vi "Create from Agent.vi"(8 "Error In":errorcluster, 11 "Agent In":refnum<class "Agent.lvclass">) -> (0 "Error Out":errorcluster, 2 "Identity":refnum<class "Agent Identity.lvclass">, 3 "Agent Out":refnum<class "Agent.lvclass">)   [LabVIEW 2018, in "Toolkit.lvlib" / "Agent Identity.lvclass"]
uses:
  Agent Identity.lvclass
  Agent/Agent.lvclass
  Agent/Agent.lvclass/Agent.ctl
  Session/Session.lvclass/Session.ctl
  SSH/SSH.lvclass
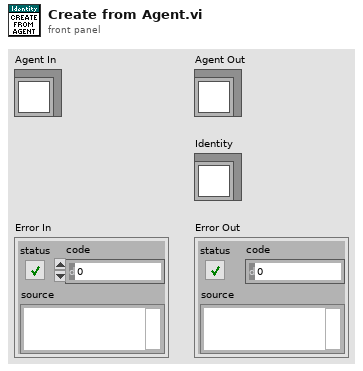
[diagram p1: front panel]
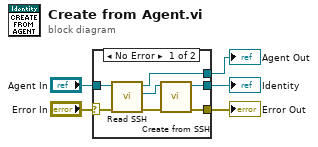
[diagram p0: block diagram]
diagram:
  n1 = case shown="No Error" "Error In" {
    selector: "Error In" -> [w7 w13]
    tunnel: "Agent In" -> [w12 w14]
    tunnel: [w11 w14] -> w3
    tunnel: [w9 _] -> w4
    tunnel: [w6 w13] -> w1
    frame No Error {
      n2 = call "Read SSH.vi"("Error In"=w7, "Agent In"=w12) -> ("Error Out"=w8:errorcluster, "SSH"=w10:refnum<class "SSH.lvclass">, "Agent Out"=w11:refnum<class "Agent.lvclass">)  [unwired: 7 in]
      n3 = call "Create from SSH.vi"("Error In"=w8, "SSH"=w10) -> ("Error Out"=w6:errorcluster, "Identity"=w9:refnum<class "Agent Identity.lvclass">)  [unwired: 8 in]
    }
    frame Error {
    }
  }
  "Identity" <- w4
  "Agent Out" <- w3
  "Error Out" <- w1
